vi "Module Identities.vi"(8 "error in (no error)":errorcluster, 11 "Event Reporter Module in":refnum<class "Event Reporter Module.lvclass">) -> (0 "error out":errorcluster, 2 "Identities":refnum<class "Identity.lvclass">[](array[class]), 3 "Event Reporter Module out":refnum<class "Event Reporter Module.lvclass">)   [LabVIEW 2020, in "Volatus.lvlib" / "Event Reporter Module.lvclass"]
uses:
  Event Reporter Module.lvclass
  Identity/Identity.lvclass
  Event Reporter Identity/Event Reporter Identity.lvclass
  C:/dev/lv20CE/relink/lv-volatus/Volatus/Identity/Identity.lvclass
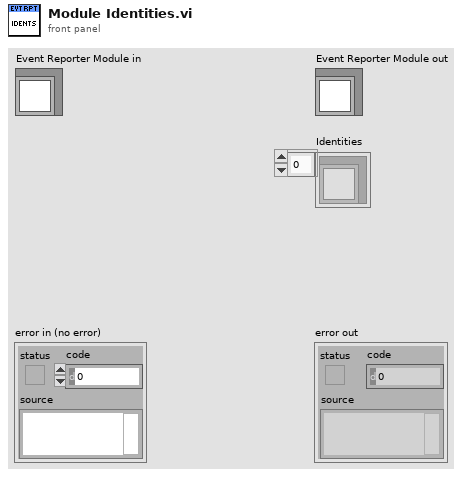
[diagram p1: front panel]
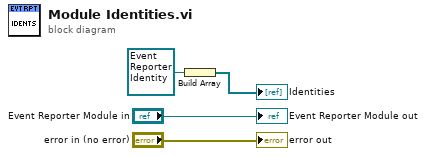
[diagram p0: block diagram]
diagram:
  n1 = Build Array(refnum<class "Event Reporter Identity.lvclass"> refnum ("Volatus:Event Reporter Identity.lvclass")) -> (→"Identities":refnum<class "Event Reporter Identity.lvclass">[])
  "error out" <- "error in (no error)"
  "Event Reporter Module out" <- "Event Reporter Module in"
